vi "NDAP_ver7.1.vi"() -> ()   [LabVIEW 2013]
panel:
  out "file path":path
  in  "stop (F)":bool
  in  "Intercepts":dbl[](array[numeric])
  in  "Slopes":dbl[](array[numeric])
  in  "Tab Control":T1(tab)
  out "PT 1":dbl[](graph)
  out "PT 2":dbl[](graph)
  out "PT 4":dbl[](graph)
  out "PT 3":dbl[](graph)
  out "PT 5":dbl[](graph)
  out "PT 6":dbl[](graph)
  out "PT 7":dbl[](graph)
  out "PT 8":dbl[](graph)
  out "LC 1":dbl[](graph)
  out "LC 2":dbl[](graph)
  out "FM":dbl[](graph)
  out "TC 1":dbl[](graph)
  out "TC 2":dbl[](graph)
  out "TC 3":dbl[](graph)
  out "TC 4":dbl[](graph)
  # "Slope must be 1 and Intercepts\nmust be 0 (not greyed out)\nfor this to work"
  # "LC Calibration"
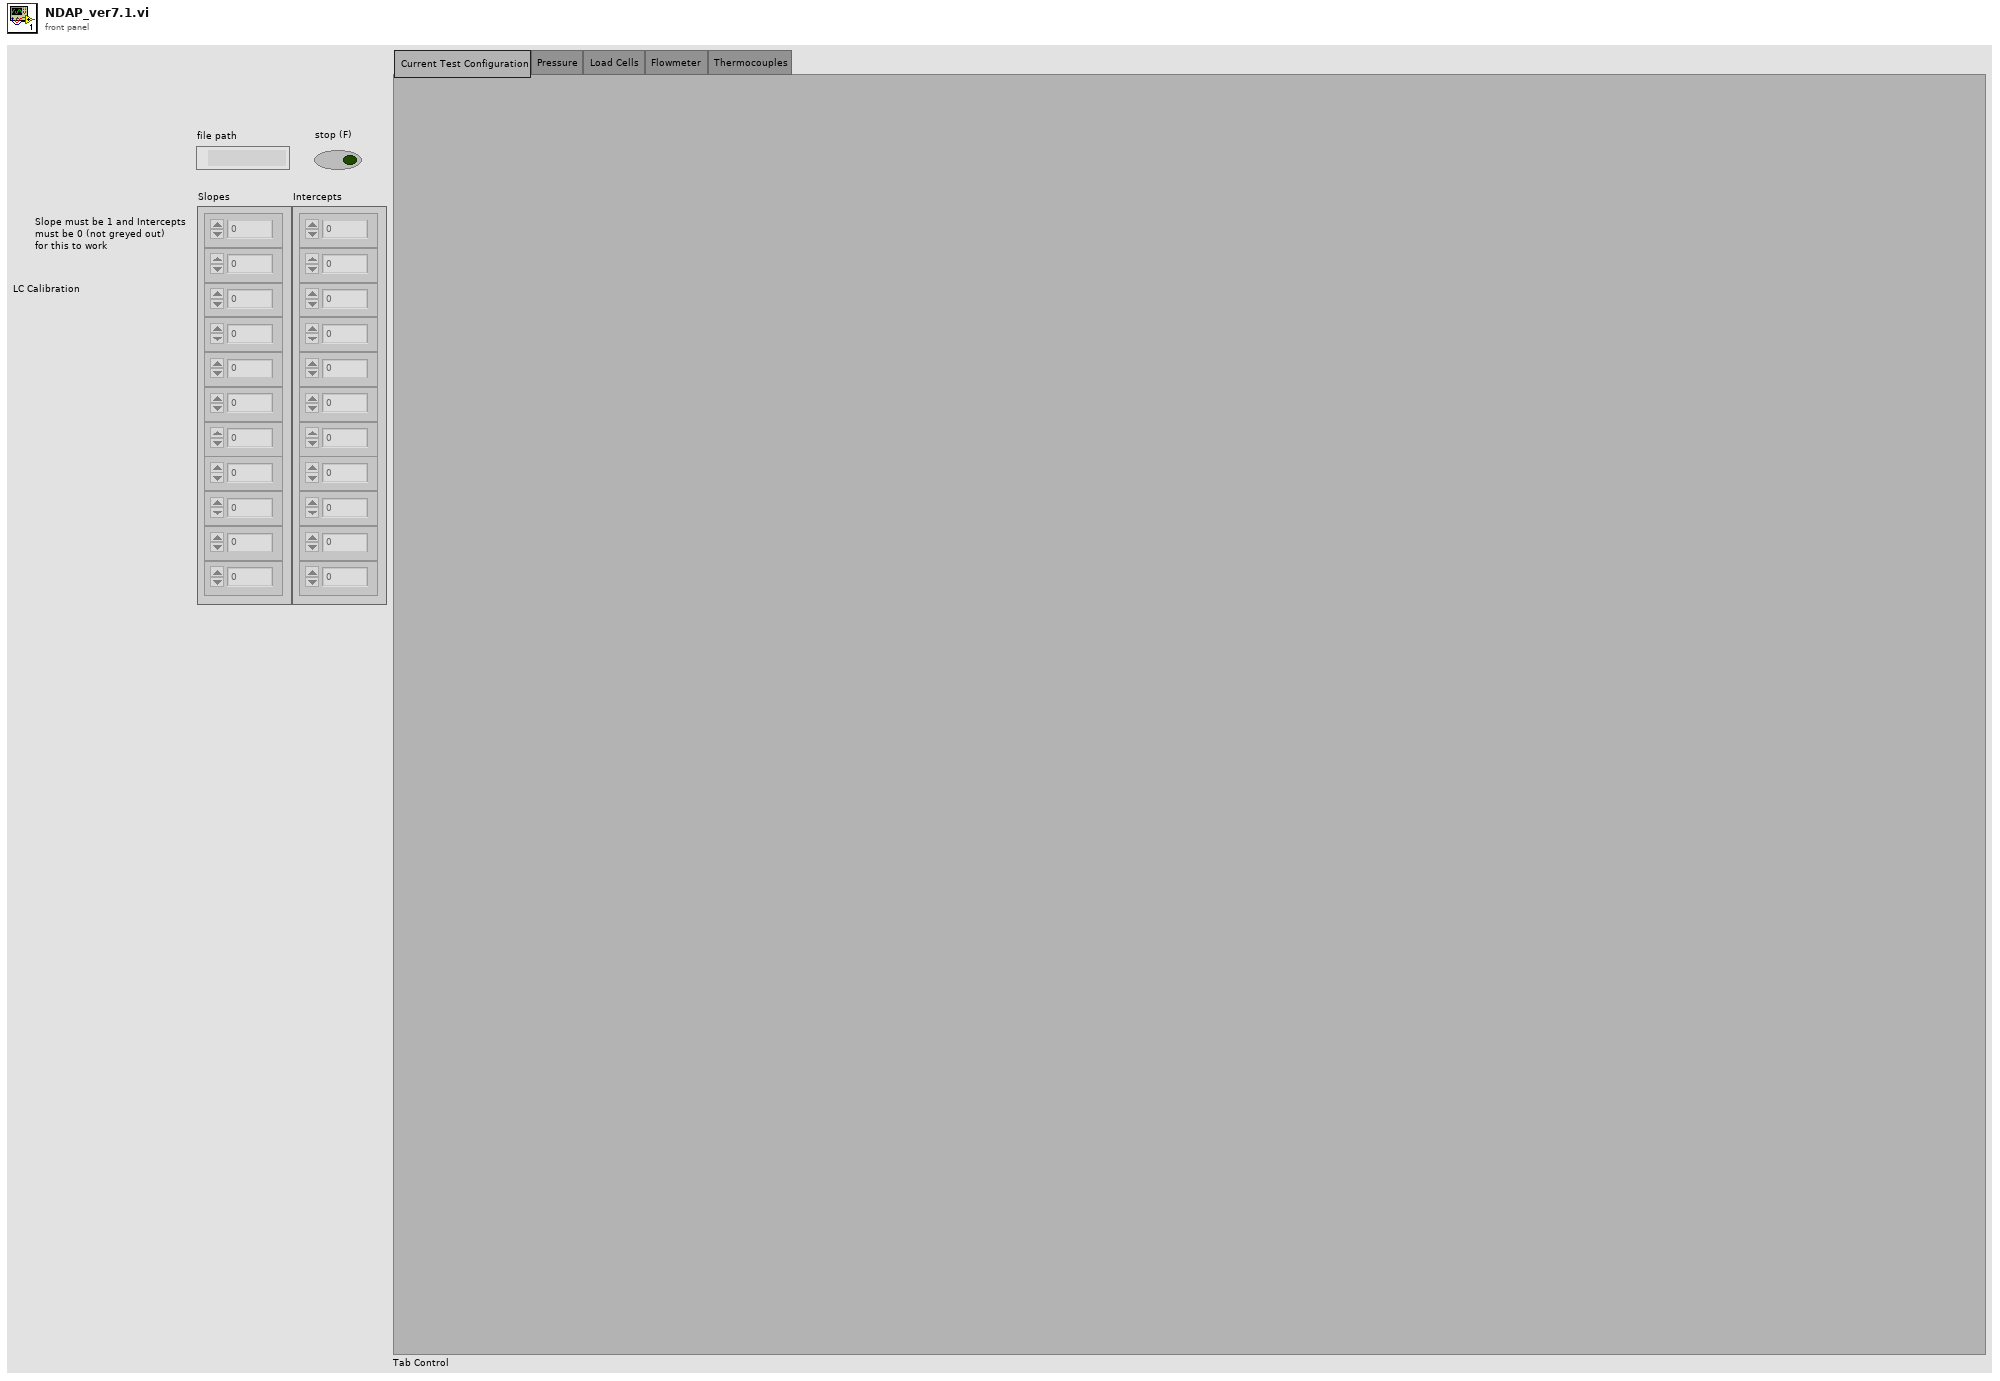
[diagram p1: front panel]
types:
  T1 = enum32{"Current Test Configuration", "Pressure", "Load Cells", "Flowmeter", "Thermocouples"}
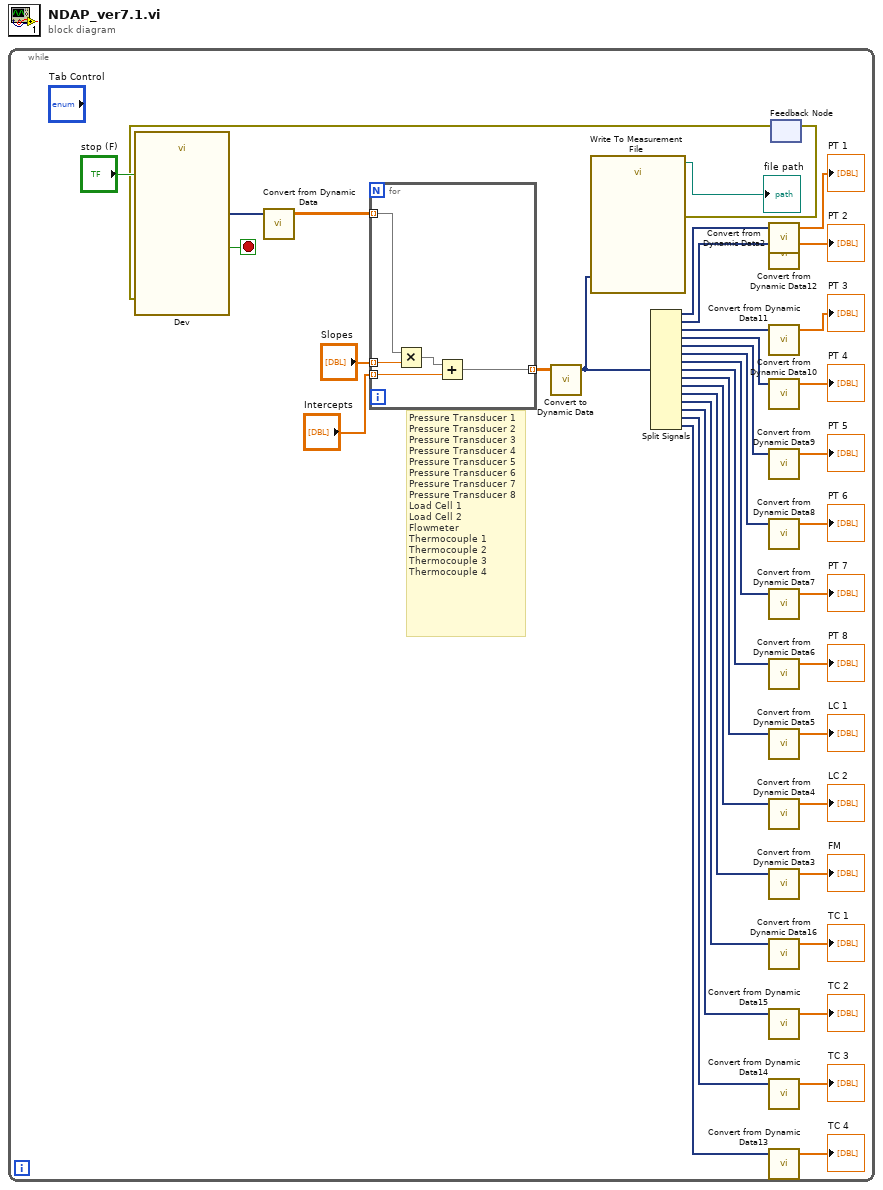
[diagram p0: block diagram]
diagram:
  n1 = while {
    stop <- w40 stop-if-true
    # "Pressure Transducer 1\nPressure Transducer 2\nPressure Transducer 3\nPressure Transducer 4\nPressure Transducer 5\nPressure Transducer 6\nPressure Transducer 7\nPressure Transducer 8\nLoad Cell 1\nLoad Cell 2\nFlowmeter\nThermocouple 1\nThermocouple 2\nThermocouple 3\nThermocouple 4"
    n2 = feedback #1() -> (w34:errorcluster)  [unwired: 1 in]
    n3 = call "Dev"("error in"=w34, "stop (F)"="stop (F)") -> ("data"=w39:dynamicdata, "stopped"=w40:bool)  [unwired: 14 in, 2 out]
    n4 = call "Convert from Dynamic Data"("Dynamic Data Type"=w39) -> ("Array"=w36:dbl[][])  [unwired: 3 in]
    n5 = for {
      tunnel: w36 -> [w46] mode=indexing
      tunnel: "Slopes" -> [w45] mode=indexing
      tunnel: "Intercepts" -> [w43] mode=indexing
      tunnel: [w42] -> w35 mode=indexing
      n6 = Multiply(x=w46, y=w45) -> (x*y=w44:dbl[])
      n7 = Add(x=w44, y=w43) -> (x+y=w42:dbl[])
    }
    n8 = call "Convert to Dynamic Data"("2D Array"=w35) -> ("Dynamic Data Type"=w5:dynamicdata)  [unwired: 3 in]
    n9 = call "Write To Measurement File"("Signals"=w5) -> ("Filename Out"=→"file path":path, "error out"=w3:errorcluster)  [unwired: 16 in, 1 out]
    n10 = Split Signals(w5) -> (w33:dynamicdata, w31:dynamicdata, w29:dynamicdata, w27:dynamicdata, w25:dynamicdata, w23:dynamicdata, w21:dynamicdata, w19:dynamicdata, w17:dynamicdata, w16:dynamicdata, w15:dynamicdata, w13:dynamicdata, w11:dynamicdata, w9:dynamicdata, w7:dynamicdata)  [unwired: 15 in]
    n11 = call "Convert from Dynamic Data2"("Dynamic Data Type"=w33) -> ("Array"=→"PT 1":dbl[])  [unwired: 3 in]
    n12 = call "Convert from Dynamic Data12"("Dynamic Data Type"=w31) -> ("Array"=→"PT 2":dbl[])  [unwired: 3 in]
    n13 = call "Convert from Dynamic Data11"("Dynamic Data Type"=w29) -> ("Array"=→"PT 3":dbl[])  [unwired: 3 in]
    n14 = call "Convert from Dynamic Data10"("Dynamic Data Type"=w27) -> ("Array"=→"PT 4":dbl[])  [unwired: 3 in]
    n15 = call "Convert from Dynamic Data9"("Dynamic Data Type"=w25) -> ("Array"=→"PT 5":dbl[])  [unwired: 3 in]
    n16 = call "Convert from Dynamic Data8"("Dynamic Data Type"=w23) -> ("Array"=→"PT 6":dbl[])  [unwired: 3 in]
    n17 = call "Convert from Dynamic Data7"("Dynamic Data Type"=w21) -> ("Array"=→"PT 7":dbl[])  [unwired: 3 in]
    n18 = call "Convert from Dynamic Data6"("Dynamic Data Type"=w19) -> ("Array"=→"PT 8":dbl[])  [unwired: 3 in]
    n19 = call "Convert from Dynamic Data5"("Dynamic Data Type"=w17) -> ("Array"=→"LC 1":dbl[])  [unwired: 3 in]
    n20 = call "Convert from Dynamic Data4"("Dynamic Data Type"=w16) -> ("Array"=→"LC 2":dbl[])  [unwired: 3 in]
    n21 = call "Convert from Dynamic Data3"("Dynamic Data Type"=w15) -> ("Array"=→"FM":dbl[])  [unwired: 3 in]
    n22 = call "Convert from Dynamic Data16"("Dynamic Data Type"=w13) -> ("Array"=→"TC 1":dbl[])  [unwired: 3 in]
    n23 = call "Convert from Dynamic Data15"("Dynamic Data Type"=w11) -> ("Array"=→"TC 2":dbl[])  [unwired: 3 in]
    n24 = call "Convert from Dynamic Data14"("Dynamic Data Type"=w9) -> ("Array"=→"TC 3":dbl[])  [unwired: 3 in]
    n25 = call "Convert from Dynamic Data13"("Dynamic Data Type"=w7) -> ("Array"=→"TC 4":dbl[])  [unwired: 3 in]
    n26 = feedback-in #1(w3) -> ()
  }
